vi "rethinkdb_msg_errors.vi"(8 "error in (no error)":errorcluster, 11 "message":string) -> (0 "error out":errorcluster)   [LabVIEW 2017]
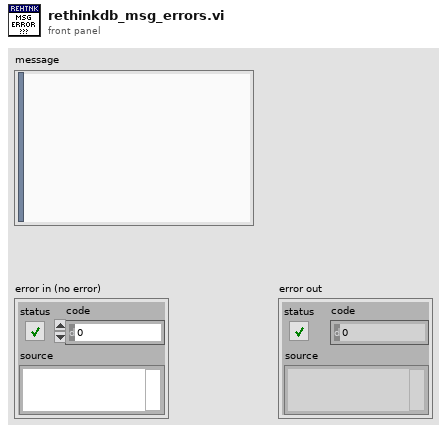
[diagram p1: front panel]
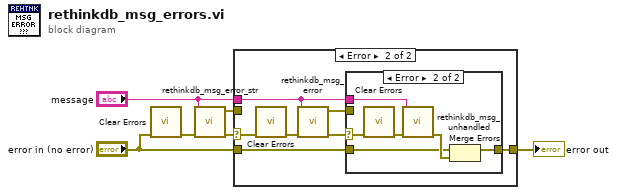
[diagram p0: block diagram]
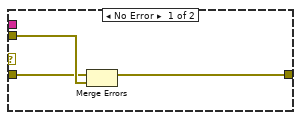
[diagram p2: hidden frame]
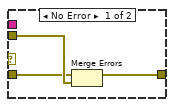
[diagram p3: hidden frame]
diagram:
  n1 = call <vilib>:"Clear Errors.vi"("error in (no error)"="error in (no error)") -> ("error out"=w2:errorcluster)  [unwired: 5 in, 1 out]
  n2 = call "rethinkdb_msg_error_str.vi"("error in (no error)"=w2, "message"="message") -> ("error out"=w6:errorcluster, "error"=w5:errorcluster)  [unwired: 8 in]
  n3 = case shown="Error" w6 {
    selector: w6 -> [_ w11]
    tunnel: "message" -> [_ w14]
    tunnel: [w9 w15] -> w3
    tunnel: w5 -> [w8 _]
    tunnel: "error in (no error)" -> [w7 w12]
    frame No Error {
      n4 = Merge Errors(w7, w8) -> (w9:errorcluster)
    }
    frame Error {
      n5 = call <vilib>:"Clear Errors.vi"("error in (no error)"=w11) -> ("error out"=w10:errorcluster)  [unwired: 5 in, 1 out]
      n6 = call "rethinkdb_msg_error.vi"("error in (no error)"=w10, "message"=w14) -> ("error out"=w16:errorcluster, "error"=w13:errorcluster)  [unwired: 8 in]
      n7 = case shown="Error" w16 {
        selector: w16 -> [_ w21]
        tunnel: [w19 w23] -> w15
        tunnel: w14 -> [_ w24]
        tunnel: w13 -> [w18 _]
        tunnel: w12 -> [w17 w22]
        frame No Error {
          n8 = Merge Errors(w17, w18) -> (w19:errorcluster)
        }
        frame Error {
          n9 = call <vilib>:"Clear Errors.vi"("error in (no error)"=w21) -> ("error out"=w20:errorcluster)  [unwired: 5 in, 1 out]
          n10 = call "rethinkdb_msg_unhandled.vi"("error in (no error)"=w20, "message"=w24) -> ("error out"=w25:errorcluster)  [unwired: 9 in]
          n11 = Merge Errors(w22, w25) -> (w23:errorcluster)
        }
      }
    }
  }
  "error out" <- w3
